vi "Read DIO Lines.vi"(8 "error in (no error)":errorcluster, 11 "RIO Target Configuration in":refnum<class "RIO Target Configuration.lvclass">) -> (0 "error out":errorcluster, 2 "DIO Lines":string[](array[string]), 3 "RIO Target Configuration out":refnum<class "RIO Target Configuration.lvclass">)   [LabVIEW 2014, in "RIO Target Configuration.lvclass"]
uses:
  RIO Target Configuration.lvclass
  <vilib>/NI/Configuration Framework/serializable configuration/NISE_CEF_serializable configuration.lvclass
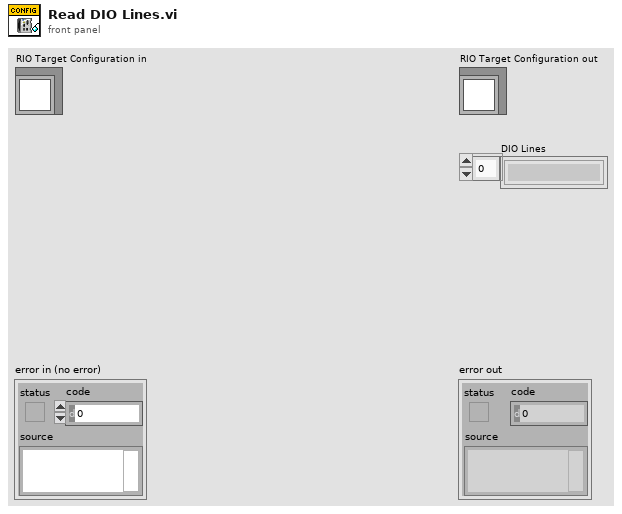
[diagram p1: front panel]
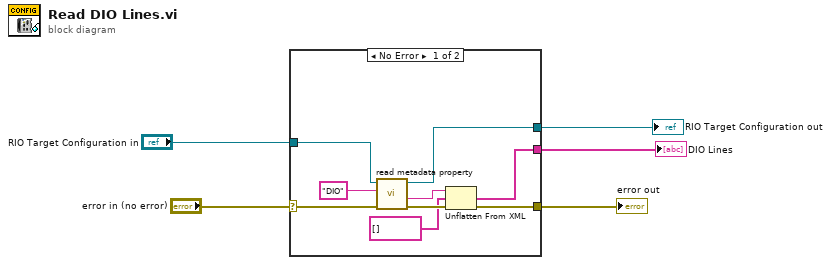
[diagram p0: block diagram]
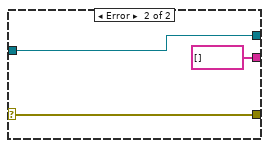
[diagram p2: hidden frame]
diagram:
  n1 = case shown="No Error" "error in (no error)" {
    selector: "error in (no error)" -> [w13 w17]
    tunnel: "RIO Target Configuration in" -> [w12 w16]
    tunnel: [w7 w17] -> w3
    tunnel: [w11 w16] -> w1
    tunnel: [w6 string[] [] ("DIO Lines")] -> w2
    frame No Error {
      n2 = call <vilib>:"read metadata property.vi"("error in"=w13, "key"="DIO", "configuration in"=w12) -> ("error out"=w10:errorcluster, "value"=w9:string, "configuration out"=w11:refnum<class "RIO Target Configuration.lvclass">)  [unwired: 5 in, 1 out]
      n3 = Unflatten From XML(xml string=w9, type=string[] [] ("DIO Lines"), error in (no error)=w10) -> (value=w6:string[], error out=w7:errorcluster)
    }
    frame Error {
    }
  }
  "error out" <- w3
  "RIO Target Configuration out" <- w1
  "DIO Lines" <- w2
